vi "resetArray (SubVI).vi"(10 "a samples in":fxp<+/-,64,32>[](array[numeric])=[0.0, 0.0, 0.0, 0.0, 0.0, 0.0, 0.0, 0.0, 0.0, 0.0, 0.0, 0.0, 0.0, 0.0, 0.0, 0.0, 0.0, 0.0, 0.0, 0.0, 0.0, 0.0, 0.0, 0.0, 0.0, 0.0, 0.0, 0.0, 0.0, 0.0, 0.0, 0.0, 0.0, 0.0, 0.0, 0.0, 0.0, 0.0, 0.0, 0.0, 0.0, 0.0, 0.0, 0.0, 0.0, 0.0, 0.0, 0.0, 0.0, 0.0]) -> (2 "a samples out":fxp<+/-,64,32>[](array[numeric]))   [LabVIEW 2017]
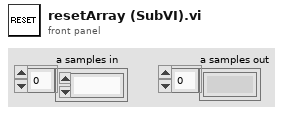
[diagram p1: front panel]
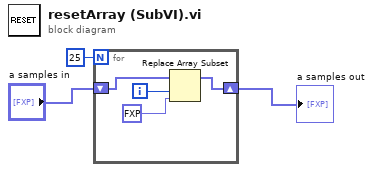
[diagram p0: block diagram]
diagram:
  n1 = for {
    N: 25 -> [_]
    shift-right: [w5] -> w2
    shift-left: "a samples in" -> [w4]
    i -> [w7]
    n2 = Replace Array Subset(array=w4, new element=fxp<+,1,2> 2.0 ("new element/subarray"), index=w7) -> (w5:fxp<+/-,64,32>[])
  }
  "a samples out" <- w2
